vi "叶绿素a_获取温度和叶绿素值.vi"(8 "error in (no error)":errorcluster caption="错误输入（无错误）", 11 "MB_Serial session in":refnum<class "MB_Master_Serial.lvclass">) -> (0 "error out":errorcluster caption="错误输出", 2 "输出值":cluster{"温度测量值":sgl, "叶绿素测量值":sgl, "错误标志":u16} {"错误标志" items=["NO Error"=0, "刷子没到位"=255]}, 3 "MB_Serial session out":refnum<class "MB_Master_Serial.lvclass">)   [LabVIEW 2016, in "斯坦道多参数.lvlib"]
uses:
  <vilib>/Plasmionique/MB Master/MB_Master_Serial/MB_Master_Serial.lvclass
  C:/Program Files (x86)/National Instruments/LabVIEW 2016/vi.lib/Plasmionique/MB Master/MB_Master/MB_Master.lvclass
  <vilib>/Plasmionique/MB Master/MB Master.lvlib
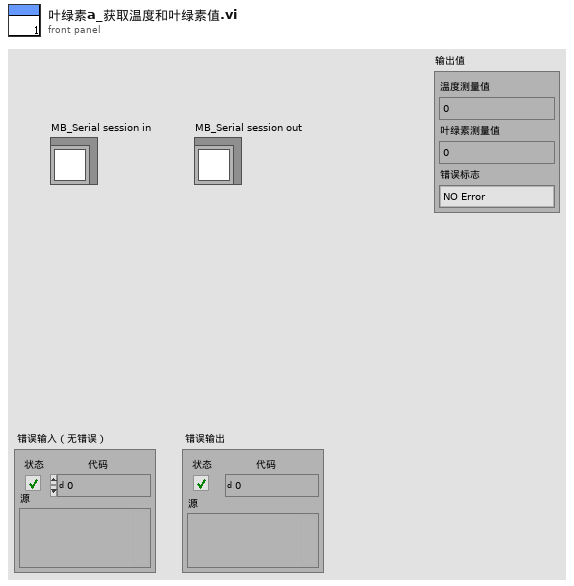
[diagram p1: front panel]
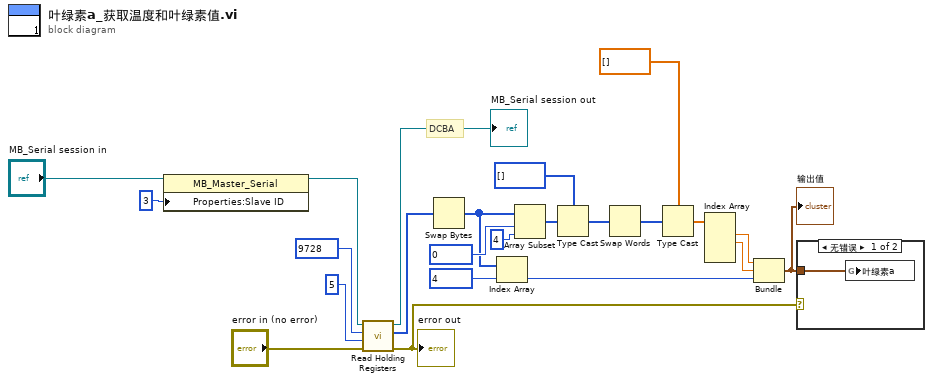
[diagram p0: block diagram]
diagram:
  # "DCBA"
  n1 = property class="MB_Master_Serial"(reference="MB_Serial session in", "Properties:Slave ID"=u16 3 ("y")) -> (reference out=w10:refnum<class "MB_Master_Serial.lvclass">)  [unwired: 1 in, 1 out]
  n2 = call <vilib>:"Read Holding Registers.vi"("error in (no error)"="error in (no error)", "quantity"=u16 5, "starting address"=u16 9728, "MB session in"=w10) -> ("error out"=w2:errorcluster, "Registers"=w5:u16[], "MB session out"=→"MB_Serial session out":refnum<class "MB_Master_Serial.lvclass">)  [unwired: 5 in]
  "error out" <- w2
  n3 = Swap Bytes(anything=w5) -> (byte swapped=w4:u16[])
  n4 = Index Array(array=w4, index=u16 4 ("starting address")) -> (element=w6:u16)
  n5 = Array Subset(array=w4, index=u16 0 ("starting address"), length=4 ("长度")) -> (w3:u16[])
  n6 = Type Cast(type=u32[] [] ("数组 2"), x=w3) -> (*(type *) &x=w17:u32[])
  n7 = Swap Words(1:w17) -> (0:w19:u32[])
  n8 = Type Cast(type=sgl[] [] ("数组 2"), x=w19) -> (*(type *) &x=w15:sgl[])
  n9 = Index Array(array=w15) -> (element #1=w14:sgl, element #2=w13:sgl)  [unwired: 4 in, 2 out]
  n10 = Bundle("数值"=w14, "数值"=w13, w6) -> (w1:cluster{"数值":sgl, "数值":sgl, u16})  [unwired: 1 in]
  "输出值" <- w1
  n11 = case shown="无错误" w2 {
    tunnel: w1 -> [w24 _]
    frame No Error {
      n12 = global write "禹山过程全局变量.vi" "叶绿素a"(w24) -> ()
    }
    frame Error {
    }
  }
